vi "Remove end of line char.vi"(8 "error in (no error)":errorcluster caption="エラー入力（エラーなし）", 11 "文字列":string="01234") -> (0 "error out":errorcluster caption="エラー出力", 3 "文字列 out":string)   [LabVIEW 2018]
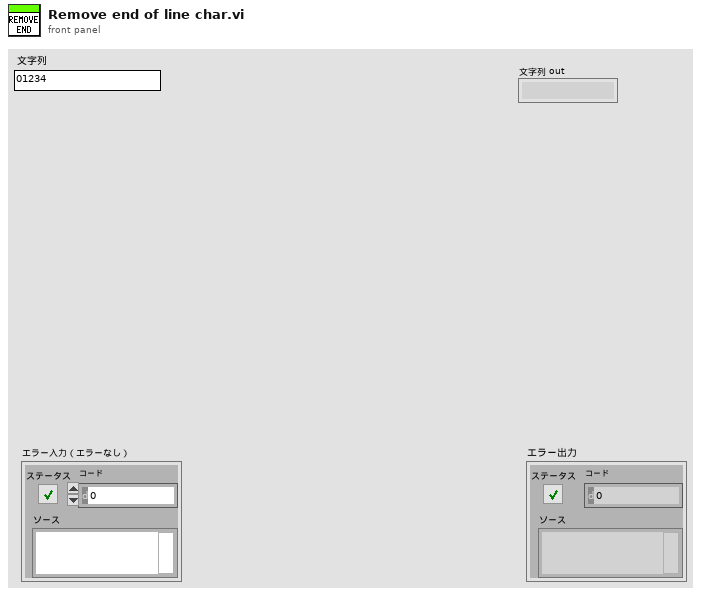
[diagram p1: front panel]
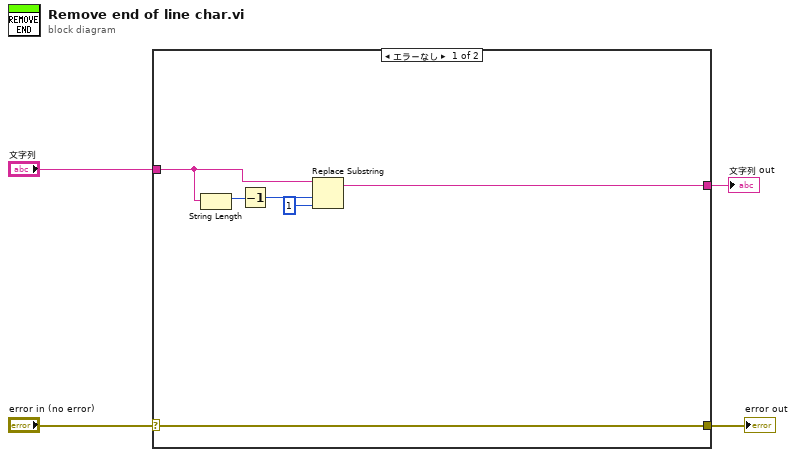
[diagram p0: block diagram]
diagram:
  n1 = case shown="エラーなし" "error in (no error)" {
    selector: "error in (no error)" -> [w10 w11]
    tunnel: [w10 w11] -> w3
    tunnel: "文字列" -> [w8 _]
    tunnel: [w5 _] -> w1
    frame No Error {
      n2 = String Length(string=w8) -> (length=w9:i32)
      n3 = Decrement(x=w9) -> (x-1=w7:i32)
      n4 = Replace Substring(2:1 ("長さ (サブ文字列の長さ)"), 3:w7, 5:w8) -> (1:w5:string)  [unwired: 1 in, 1 out]
    }
    frame Error {
    }
  }
  "error out" <- w3
  "文字列 out" <- w1
